vi "TDMS chan to HDF5 (u64).vi"(0 "tdms file":refnum<k34>, 1 "close dataset? (T)":bool=TRUE, 5 "group name in":string, 7 "channel name in":string, 11 "error in (no error)":errorcluster, 13 "HDF5 Ref":T1) -> (4 "tdms file out":refnum<k34>, 6 "group name out":string, 8 "channel name out":string, 10 "dataset out":T1, 15 "error out":errorcluster)   [LabVIEW 2012]
uses:
  <vilib>/addons/_hdf5/library.llb/HDF5 Ref.ctl
  <vilib>/addons/_hdf5/dataspace.llb/H5S_seloper_t.ctl
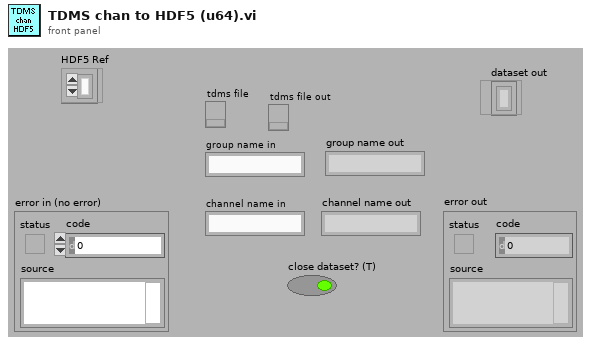
[diagram p1: front panel]
types:
  T1 = typedef "HDF5 Ref.ctl" = refnum<k1>
  T2 = typedef "H5S_seloper_t.ctl" = i32
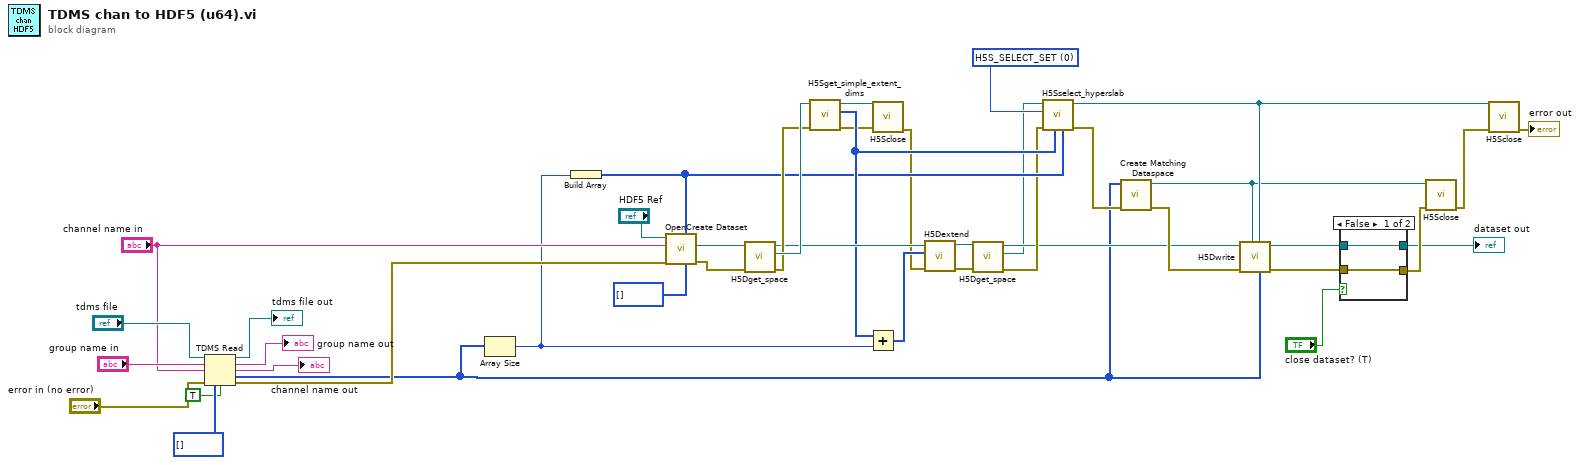
[diagram p0: block diagram]
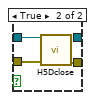
[diagram p2: hidden frame]
diagram:
  w31 = T2 0 items=["H5S_SELECT_NOOP"=-1, "H5S_SELECT_SET"=0, "H5S_SELECT_OR"=1, "H5S_SELECT_AND"=2, "H5S_SELECT_XOR"=3, "H5S_SELECT_NOTB"=4, "H5S_SELECT_NOTA"=5, "H5S_SELECT_APPEND"=6, "H5S_SELECT_PREPEND"=7] ("Operator")
  n1 = TDMS Read(0:"tdms file", 5:"group name in", 7:"channel name in", 11:"error in (no error)", 12:u64[] [], 13:TRUE ("return channels in file order? (F)")) -> (4:→"tdms file out":refnum<k34>, 6:→"group name out":string, 8:→"channel name out":string, 10:w2:u64[], 15:w37:errorcluster)  [unwired: 2 in, 1 out]
  n2 = Array Size(array=w2) -> (size(s)=w16:i32)
  n3 = Build Array(w16) -> (w15:i32[])
  n4 = call "OpenCreate Dataset.vi"("Datatype"=i16[] [], "Chunk size"=w15, "error in (no error)"=w37, "Dataset Path"="channel name in", "HDF5 Ref"="HDF5 Ref") -> ("error out"=w36:errorcluster, "HDF5 Dataset Ref out"=w28:T1)  [unwired: 4 in, 1 out]
  n5 = call <vilib>:"H5Dget_space.vi"("error in (no error)"=w36, "HDF5 Dataset Ref"=w28) -> ("error out"=w34:errorcluster, "HDF5 Dataspace Ref"=w35:T1, "HDF5 Dataset Ref out"=w32:T1)  [unwired: 5 in]
  n6 = call <vilib>:"H5Sget_simple_extent_dims.vi"("error in (no error)"=w34, "HDF5 Space Ref"=w35) -> ("error out"=w14:errorcluster, "Dims"=w30:i32[], "HDF5 Ref out"=w13:T1)  [unwired: 4 in, 1 out]
  n7 = Add(x=w30, y=w16) -> (x+y=w33:i32[])
  n8 = call <vilib>:"H5Sclose.vi"("error in (no error)"=w14, "HDF5 Dataspace Ref"=w13) -> ("error out"=w10:errorcluster)  [unwired: 7 in]
  n9 = call <vilib>:"H5Dextend.vi"("error in (no error)"=w10, "Size"=w33, "HDF5 Dataset Ref"=w32) -> ("error out"=w11:errorcluster, "HDF5 Dataset Ref out"=w12:T1)  [unwired: 5 in]
  n10 = call <vilib>:"H5Dget_space.vi"("error in (no error)"=w11, "HDF5 Dataset Ref"=w12) -> ("error out"=w9:errorcluster, "HDF5 Dataspace Ref"=w7:T1, "HDF5 Dataset Ref out"=w8:T1)  [unwired: 5 in]
  n11 = call <vilib>:"H5Sselect_hyperslab.vi"("Count"=w15, "Start"=w30, "error in (no error)"=w9, "Operator"=w31, "HDF5 Space Ref"=w7) -> ("error out"=w29:errorcluster, "HDF5 Ref out"=w24:T1)  [unwired: 5 in]
  n12 = call <vilib>:"Create Matching Dataspace.vi"("error in (no error)"=w29, "Data"=w2) -> ("error out"=w27:errorcluster, "HDF5 Dataspace Ref"=w23:T1)  [unwired: 6 in]
  n13 = call <vilib>:"H5Dwrite.vi"("Variant"=w2, "HDF5 File Space Ref (H5S_ALL)"=w24, "HDF5 Memory Space Ref (H5S_ALL)"=w23, "error in (no error)"=w27, "HDF5 Dataset Ref"=w8) -> ("error out"=w25:errorcluster, "HDF5 Ref out"=w26:T1)  [unwired: 5 in]
  n14 = case shown="False" "close dataset? (T)" {
    tunnel: w26 -> [w44 w47]
    tunnel: w25 -> [w43 w46]
    tunnel: [w43 w45] -> w22
    tunnel: [w44 _] -> w3
    frame False {
    }
    frame True {
      n15 = call <vilib>:"H5Dclose.vi"("error in (no error)"=w46, "HDF5 Dataset Ref"=w47) -> ("error out"=w45:errorcluster)  [unwired: 7 in]
    }
  }
  "dataset out" <- w3
  n16 = call <vilib>:"H5Sclose.vi"("error in (no error)"=w22, "HDF5 Dataspace Ref"=w23) -> ("error out"=w21:errorcluster)  [unwired: 7 in]
  n17 = call <vilib>:"H5Sclose.vi"("error in (no error)"=w21, "HDF5 Dataspace Ref"=w24) -> ("error out"=→"error out":errorcluster)  [unwired: 7 in]
